vi "Launch View.vi"(8 "error in (no error)":errorcluster, 9 "UUID":string, 10 "Controller in":refnum<class "Controller.lvclass">, 11 "UI View in":refnum<class "UI View.lvclass">) -> (0 "error out":errorcluster, 3 "Caller-To-Actor Enqueuer":refnum<class "Message Enqueuer.lvclass">)   [LabVIEW 2013, in "SET Project Editor.lvlib" / "UI View.lvclass"]
uses:
  UI View.lvclass
  Controller/Controller.lvclass
  <vilib>/ActorFramework/Message Enqueuer/Message Enqueuer.lvclass
  <vilib>/ActorFramework/Actor/Actor.lvclass/Actor.ctl
  <vilib>/ActorFramework/Message Enqueuer/Message Enqueuer.lvclass/Message Enqueuer.ctl
  UI View.lvclass/UI View.ctl
  <vilib>/ActorFramework/Message Enqueuer/Init from Existing Queue.vi
  <vilib>/ActorFramework/Actor/Actor.lvclass
panel:
  # "This is the view launcher.\nIt is used to setup the view with initial values from\nthe controller and to launch the view.\nThis VI is meant to be run by the controller's \"actor core.vi\".\nThe view's Caller-To-Actor Enqueuer is passed back to the controller."
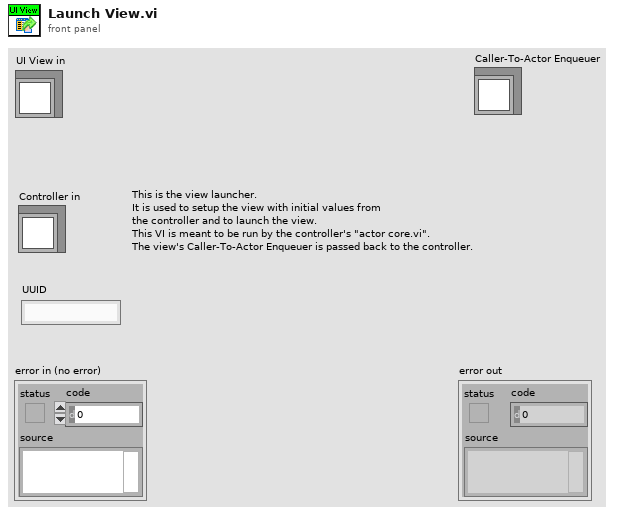
[diagram p1: front panel]
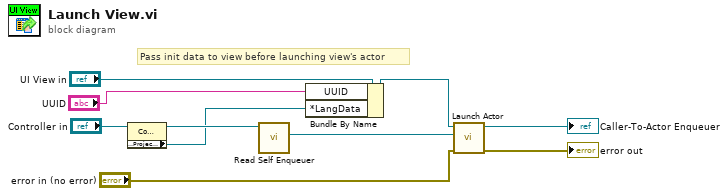
[diagram p0: block diagram]
diagram:
  # "Pass init data to view before launching view's actor"
  n1 = property class="Controller.lvclass"(reference="Controller in") -> (reference out=w3:refnum<class "Controller.lvclass">, "Properties:Project Data ref"=w2:refnum<data-value>)  [unwired: 1 in, 1 out]
  n2 = call <vilib>:"Read Self Enqueuer.vi"("Actor"=w3) -> ("Self Enqueuer"=w10:refnum<class "Message Enqueuer.lvclass">)  [unwired: 10 in]
  n3 = Bundle By Name(cluster="UI View in", "UUID"="UUID", "*LangData"=w2) -> (w5:refnum<class "UI View.lvclass">)
  n4 = call <vilib>:"Launch Actor.vi"("error in (no error)"="error in (no error)", "Actor-to-Caller Enqueuer"=w10, "Actor"=w5) -> ("error out"=→"error out":errorcluster, "Caller-To-Actor Enqueuer"=→"Caller-To-Actor Enqueuer":refnum<class "Message Enqueuer.lvclass">)  [unwired: 7 in]
